vi "Swap Data.vi"(8 "error in (no error)":errorcluster, 10 "New Data":refnum<class "Data.lvclass">, 11 "Old Data":refnum<class "Data.lvclass">) -> (0 "error out":errorcluster, 3 "Data out":refnum<class "Data.lvclass">)   [LabVIEW 2014, in "Base Data Class.lvlib" / "Data.lvclass"]
uses:
  Data.lvclass
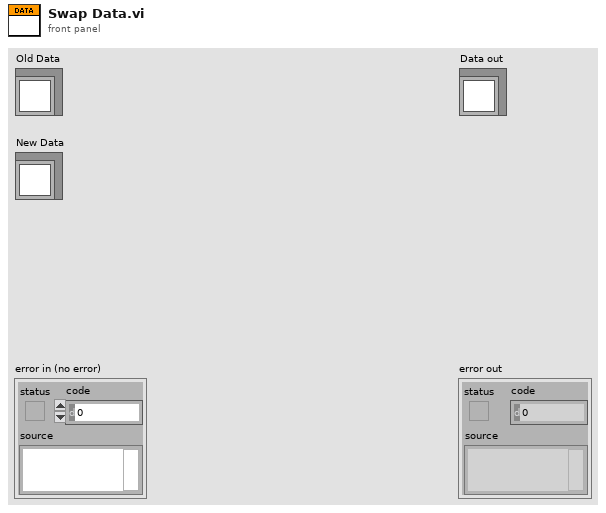
[diagram p1: front panel]
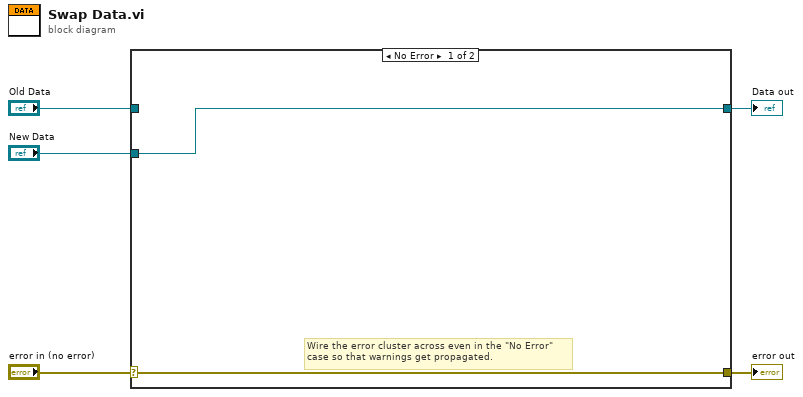
[diagram p0: block diagram]
diagram:
  n1 = case shown="No Error" "error in (no error)" {
    selector: "error in (no error)" -> [w7 w9]
    tunnel: [w7 w9] -> w4
    tunnel: [w6 w8] -> w2
    tunnel: "Old Data" -> [_ w8]
    tunnel: "New Data" -> [w6 _]
    frame No Error {
      # "Wire the error cluster across even in the \"No Error\"\ncase so that warnings get propagated."
    }
    frame Error {
    }
  }
  "error out" <- w4
  "Data out" <- w2
